vi "AMC_QuickMovePan.vi"(8 "error in (no error)":errorcluster caption="entrée d'erreur (pas d'erreur)", 11 "ConnID":refnum<k5>) -> (0 "error out":errorcluster caption="sortie d'erreur")   [LabVIEW 2019]
uses:
  <vilib>/Utility/config.llb/Read Key (String).vi
  <vilib>/Utility/config.llb/Read Key (U32).vi
  <vilib>/Utility/config.llb/NI_LVConfig.lvlib
panel:
  in  "Ctrl 3":bool
  in  "Ctrl 2":bool
  in  "Ctrl1":bool
  in  "Step3(um)":dbl=0.25 caption="Focus Step(um)"
  in  "Step2(um)":dbl=1.0 caption="Y Step(um)"
  in  "Axis Nm 1":string
  in  "axis3":u8
  in  "Init":bool
  in  "axis1":u8
  in  "axis2":u8
  in  "Axis Nm 3":string
  in  "Axis Nm 2":string
  in  "Up Z":bool
  in  "Down Z":bool
  in  "Quit":bool
  in  "Target 3":dbl=60.0 caption="Focus Target(um)" min=-25000.0 max=25000.0 step=0.001 format="%#.3f"
  out "ActPos 3":dbl=60.0 caption="Focus Act. Pos(um)" min=0.1 step=0.1 format="%#.3f"
  out "ActPos 2":dbl=60.0 caption="Y Act. Pos(um)" min=0.1 step=0.1 format="%#.3f"
  in  "Target 2":dbl=60.0 caption="Y Target(um)" min=-25000.0 max=25000.0 step=0.001 format="%#.3f"
  in  "Target 1":dbl=60.0 caption="X Target(um)" min=-25000.0 max=25000.0 step=0.001 format="%#.3f"
  out "ActPos":dbl=60.0 caption="X Act. Pos(um)" min=0.1 step=0.1 format="%#.3f"
  in  "Right":bool
  in  "Left":bool
  in  "Step1(um)":dbl=1.0 caption="X Step(um)"
  in  "Down":bool
  in  "Up":bool
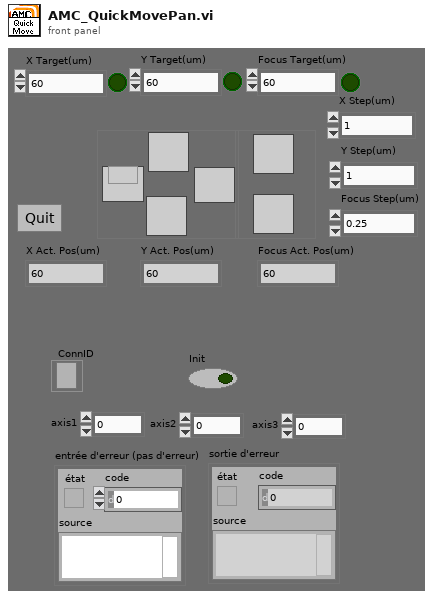
[diagram p1: front panel]
types:
  T1 = enum16{"Répertoire du VI actuel", "Répertoire du parent 1", "Répertoire du parent 2", "Répertoire du parent 3"}
  T2 = typedef "NI_LVConfig.lvlib/Config Data RefNum.ctl" = refnum<k1>
  T3 = typedef "LVRectTypeDef.ctl" = cluster{"Left":i16, "Top":i16, "Right":i16, "Bottom":i16}
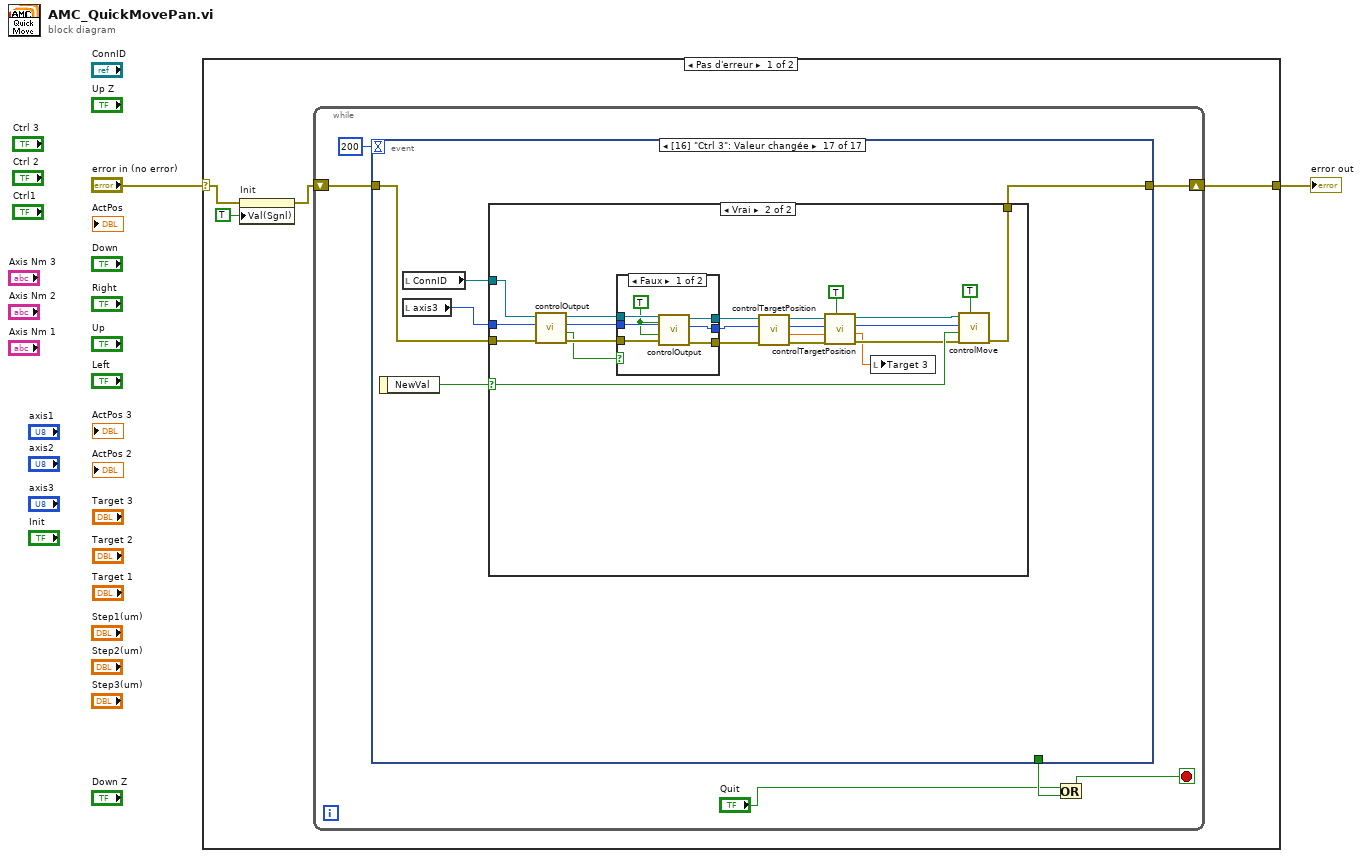
[diagram p0: block diagram]
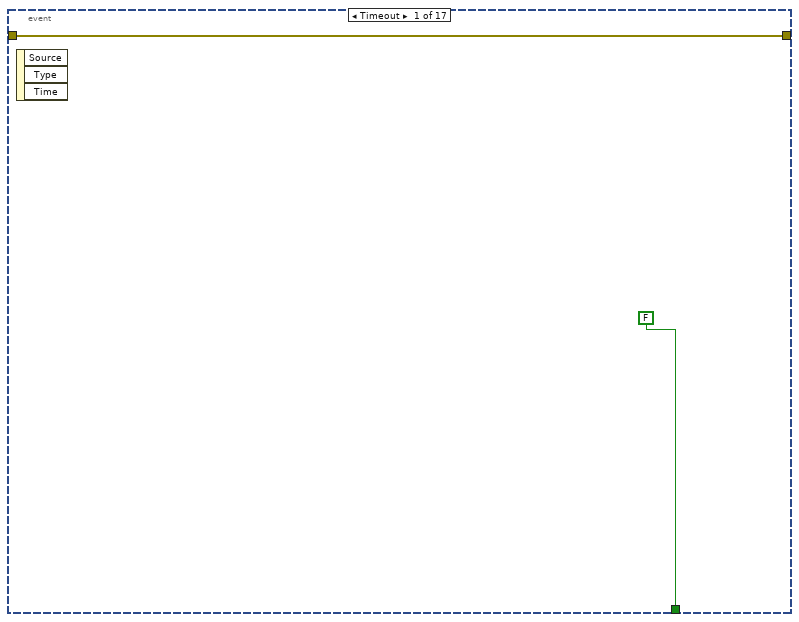
[diagram p2: hidden frame]
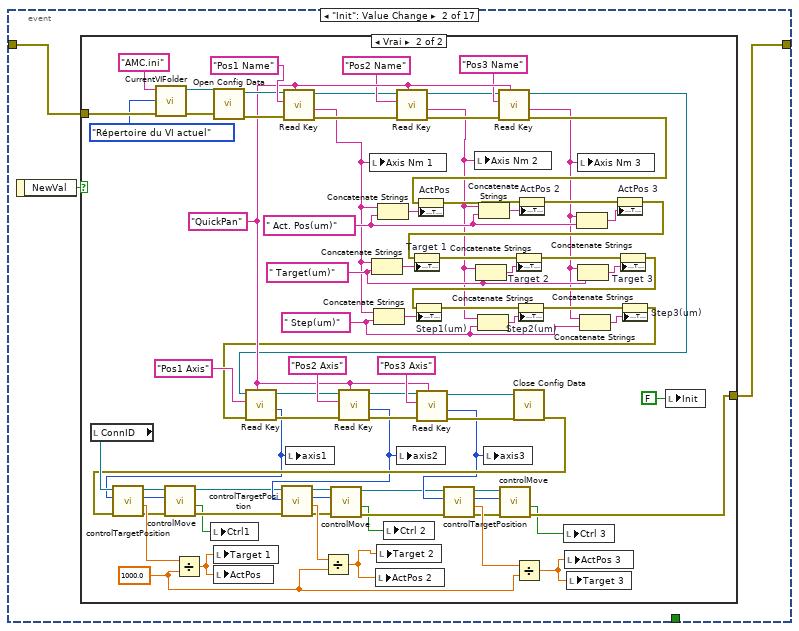
[diagram p3: hidden frame]
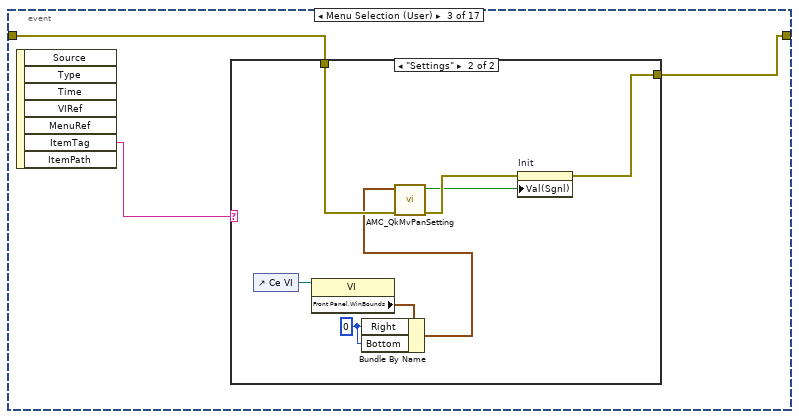
[diagram p5: hidden frame]
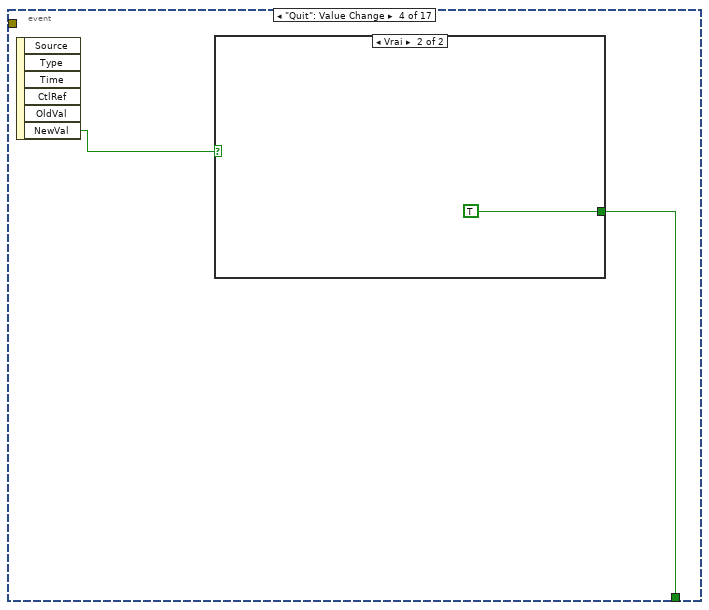
[diagram p7: hidden frame]
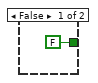
[diagram p8: hidden frame]
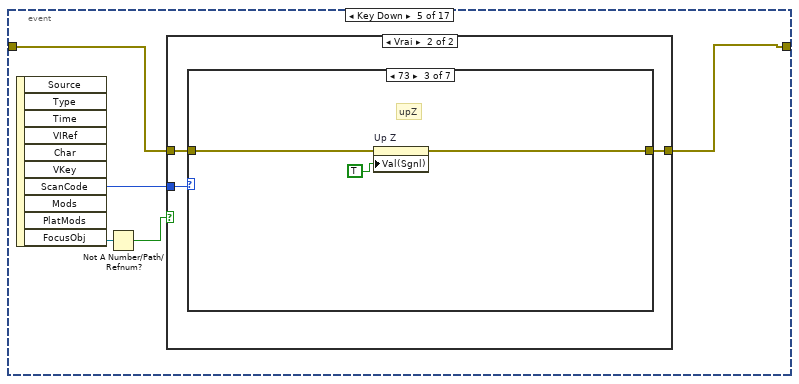
[diagram p9: hidden frame]
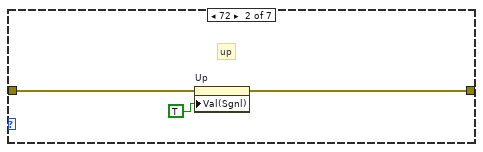
[diagram p12: hidden frame]
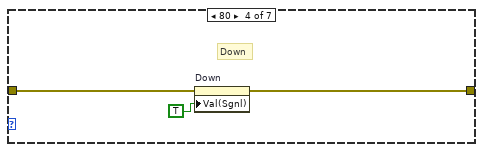
[diagram p13: hidden frame]
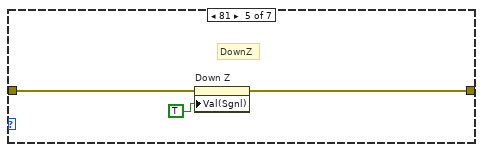
[diagram p14: hidden frame]
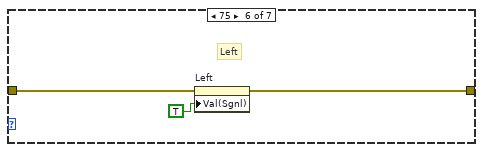
[diagram p15: hidden frame]
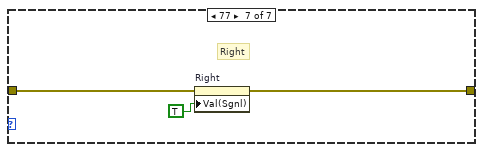
[diagram p16: hidden frame]
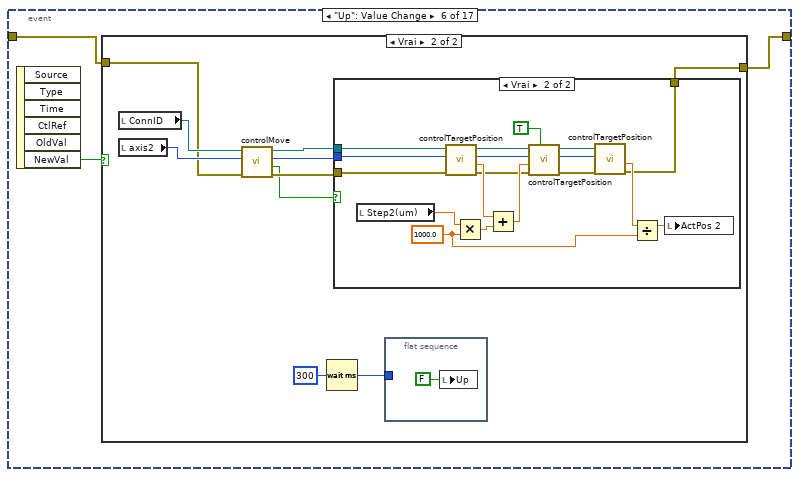
[diagram p17: hidden frame]
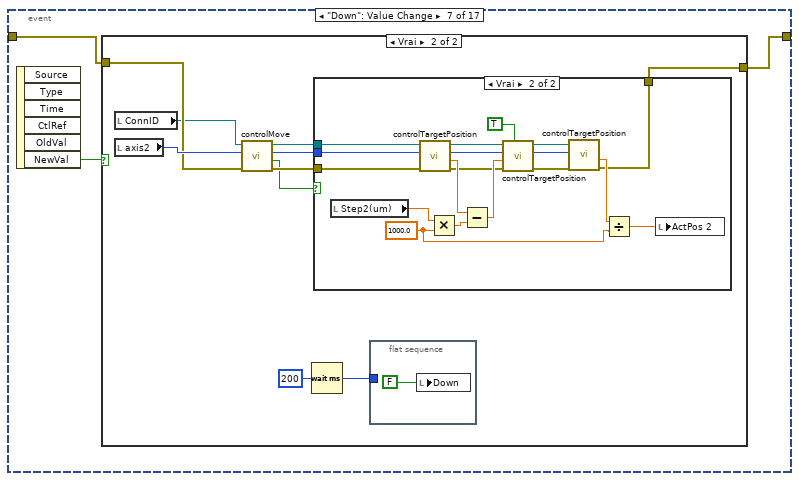
[diagram p20: hidden frame]
diagram:
  n1 = case shown="Pas d'erreur" "error in (no error)" {
    selector: "error in (no error)" -> [w5 w552]
    tunnel: [w6 w552] -> w2
    frame No Error {
      n2 = property on="Init" class="Bool (strict)"(error in=w5, "Val(Sgnl)"=TRUE ("Valeur (Signalisation)")) -> (error out=w4:errorcluster)  [unwired: 1 in, 1 out]
      n3 = while {
        shift-right: [w11] -> w6
        shift-left: w4 -> [w10]
        stop <- w8 stop-if-true
        n4 = event shown="[16] \"Ctrl 3\": Valeur changée" {
          selector: _ -> [_ _ _ _ _ _ _ _ _ _ _ _ _ _ _ _ _]
          dyn-events: _ -> [_ _ _ _ _ _ _ _ _ _ _ _ _ _ _ _ _]
          timeout: 200 -> [_ _ _ _ _ _ _ _ _ _ _ _ _ _ _ _ _]
          tunnel: [w14 w15 w99 _ w118 w143 w177 w211 w245 w279 w313 w356 w382 w407 w423 w466 w509] -> w11
          tunnel: w10 -> [w14 w16 w100 _ w119 w144 w178 w212 w246 w280 w314 w353 w378 w405 w424 w467 w510]
          tunnel: [FALSE _ _ w111 _ _ _ _ _ _ _ _ _ _ _ _ _] -> w9
          event Timeout {
            n5 = event-data() -> ()  [unwired: 1 in, 3 out]
          }
          event "Init": Value Change {
            n6 = event-data() -> ("NewVal"=w17:bool)  [unwired: 1 in]
            n7 = case shown="Vrai" w17 {
              tunnel: w16 -> [w18 w90]
              tunnel: [w18 w22] -> w15
              frame False {
              }
              frame True {
                w42 = 1000.0 ("y")
                w58 = " Step(um)" ("key")
                w59 = " Target(um)" ("key")
                w69 = " Act. Pos(um)" ("key")
                w84 = "QuickPan" ("section")
                n8 = local read "ConnID"() -> (w47:refnum<k5>)
                n9 = call <userlib>:"CurrentVIFolder.vi"("error in (no error)"=w90, "Source"=T1."Répertoire du VI actuel", "NomFichier"="AMC.ini") -> ("error out"=w91:errorcluster, "Chemin"=w92:path)  [unwired: 6 in, 1 out]
                n10 = call <vilib>:"Open Config Data.vi"("error in (no error)"=w91, "configuration file path"=w92) -> ("error out"=w87:errorcluster, "refnum"=w93:T2)  [unwired: 7 in, 1 out]
                n11 = call-poly <vilib>:"Read Key.vi"("section"=w84, "error in (no error)"=w87, "key"="Pos1 Name", "refnum"=w93) -> ("error out"=w86:errorcluster, "value"=w50:string, "refnum out"=w73:T2)  [unwired: 4 in, 1 out]
                n12 = local write "Axis Nm 1"(w50) -> ()
                n13 = Concatenate Strings(w50, w59) -> (w61:string)
                n14 = Concatenate Strings(w50, w58) -> (w57:string)
                n15 = Concatenate Strings(w50, w69) -> (w72:string)
                n16 = call-poly <vilib>:"Read Key.vi"("section"=w84, "error in (no error)"=w86, "key"="Pos2 Name", "refnum"=w73) -> ("error out"=w85:errorcluster, "value"=w49:string, "refnum out"=w74:T2)  [unwired: 4 in, 1 out]
                n17 = local write "Axis Nm 2"(w49) -> ()
                n18 = Concatenate Strings(w49, w59) -> (w62:string)
                n19 = Concatenate Strings(w49, w58) -> (w56:string)
                n20 = Concatenate Strings(w49, w69) -> (w71:string)
                n21 = call-poly <vilib>:"Read Key.vi"("section"=w84, "error in (no error)"=w85, "key"="Pos3 Name", "refnum"=w74) -> ("error out"=w68:errorcluster, "value"=w48:string, "refnum out"=w75:T2)  [unwired: 4 in, 1 out]
                n22 = property on="ActPos" class="NumNb (strict)"(error in=w68, "Caption.Text"=w72) -> (error out=w67:errorcluster)  [unwired: 1 in, 1 out]
                n23 = property on="ActPos 2" class="NumNb (strict)"(error in=w67, "Caption.Text"=w71) -> (error out=w66:errorcluster)  [unwired: 1 in, 1 out]
                n24 = Concatenate Strings(w48, w69) -> (w70:string)
                n25 = local write "Axis Nm 3"(w48) -> ()
                n26 = Concatenate Strings(w48, w59) -> (w63:string)
                n27 = Concatenate Strings(w48, w58) -> (w55:string)
                n28 = property on="ActPos 3" class="NumNb (strict)"(error in=w66, "Caption.Text"=w70) -> (error out=w60:errorcluster)  [unwired: 1 in, 1 out]
                n29 = property on="Target 1" class="NumNb (strict)"(error in=w60, "Caption.Text"=w61) -> (error out=w64:errorcluster)  [unwired: 1 in, 1 out]
                n30 = property on="Target 2" class="NumNb (strict)"(error in=w64, "Caption.Text"=w62) -> (error out=w65:errorcluster)  [unwired: 1 in, 1 out]
                n31 = property on="Target 3" class="NumNb (strict)"(error in=w65, "Caption.Text"=w63) -> (error out=w51:errorcluster)  [unwired: 1 in, 1 out]
                n32 = property on="Step1(um)" class="NumNb (strict)"(error in=w51, "Caption.Text"=w57) -> (error out=w54:errorcluster)  [unwired: 1 in, 1 out]
                n33 = property on="Step2(um)" class="NumNb (strict)"(error in=w54, "Caption.Text"=w56) -> (error out=w53:errorcluster)  [unwired: 1 in, 1 out]
                n34 = property on="Step3(um)" class="NumNb (strict)"(error in=w53, "Caption.Text"=w55) -> (error out=w52:errorcluster)  [unwired: 1 in, 1 out]
                n35 = call-poly <vilib>:"Read Key.vi"("section"=w84, "error in (no error)"=w52, "key"="Pos1 Axis", "refnum"=w75) -> ("error out"=w77:errorcluster, "value"=w39:u32, "refnum out"=w81:T2)  [unwired: 4 in, 1 out]
                n36 = local write "axis1"(w39) -> ()
                n37 = call-poly <vilib>:"Read Key.vi"("section"=w84, "error in (no error)"=w77, "key"="Pos2 Axis", "refnum"=w81) -> ("error out"=w76:errorcluster, "value"=w38:u32, "refnum out"=w80:T2)  [unwired: 4 in, 1 out]
                n38 = local write "axis2"(w38) -> ()
                n39 = call-poly <vilib>:"Read Key.vi"("section"=w84, "error in (no error)"=w76, "key"="Pos3 Axis", "refnum"=w80) -> ("error out"=w78:errorcluster, "value"=w37:u32, "refnum out"=w79:T2)  [unwired: 4 in, 1 out]
                n40 = local write "axis3"(w37) -> ()
                n41 = call <vilib>:"Close Config Data.vi"("error in (no error)"=w78, "refnum"=w79) -> ("error out"=w46:errorcluster)  [unwired: 8 in, 1 out]
                n42 = call <userlib>:"controlTargetPosition.vi"("error in"=w46, "axis in"=w39, "connection ID"=w47) -> ("error out"=w34:errorcluster, "Target Position out"=w36:dbl, "axis out"=w33:u8, "connection ID"=w35:refnum<k5>)  [unwired: 5 in]
                n43 = call <userlib>:"controlMove.vi"("error in"=w34, "axis in"=w33, "connection ID"=w35) -> ("error out"=w26:errorcluster, "controll move out"=w21:bool, "connection ID"=w25:refnum<k5>)  [unwired: 5 in, 1 out]
                n44 = Divide(x=w36, y=w42) -> (x/y=w44:dbl)
                n45 = local write "Ctrl1"(w21) -> ()
                n46 = local write "Target 1"(w44) -> ()
                n47 = local write "ActPos"(w44) -> ()
                n48 = call <userlib>:"controlTargetPosition.vi"("error in"=w26, "axis in"=w38, "connection ID"=w25) -> ("error out"=w32:errorcluster, "Target Position out"=w45:dbl, "axis out"=w30:u8, "connection ID"=w31:refnum<k5>)  [unwired: 5 in]
                n49 = Divide(x=w45, y=w42) -> (x/y=w43:dbl)
                n50 = call <userlib>:"controlMove.vi"("error in"=w32, "axis in"=w30, "connection ID"=w31) -> ("error out"=w23:errorcluster, "controll move out"=w19:bool, "connection ID"=w24:refnum<k5>)  [unwired: 5 in, 1 out]
                n51 = local write "ActPos 2"(w43) -> ()
                n52 = local write "Target 2"(w43) -> ()
                n53 = local write "Ctrl 2"(w19) -> ()
                n54 = call <userlib>:"controlTargetPosition.vi"("error in"=w23, "axis in"=w37, "connection ID"=w24) -> ("error out"=w29:errorcluster, "Target Position out"=w41:dbl, "axis out"=w27:u8, "connection ID"=w28:refnum<k5>)  [unwired: 5 in]
                n55 = call <userlib>:"controlMove.vi"("error in"=w29, "axis in"=w27, "connection ID"=w28) -> ("error out"=w22:errorcluster, "controll move out"=w20:bool)  [unwired: 5 in, 2 out]
                n56 = Divide(x=w41, y=w42) -> (x/y=w40:dbl)
                n57 = local write "Ctrl 3"(w20) -> ()
                n58 = local write "ActPos 3"(w40) -> ()
                n59 = local write "Target 3"(w40) -> ()
                n60 = local write "Init"(FALSE ("Init")) -> ()
              }
            }
          }
          event Menu Selection (User) {
            n61 = event-data() -> ("ItemTag"=w101:string)  [unwired: 1 in, 6 out]
            n62 = case shown="\"Settings\"" w101 {
              tunnel: w100 -> [w102 w109]
              tunnel: [w102 w110] -> w99
              frame Default {
              }
              frame "Settings" {
                w104 = i16 0 ("Right")
                n63 = control-ref of="Ce VI"() -> (w106:refnum<vi>)
                n64 = property class="VI"(reference=w106) -> ("Front Panel.WinBounds"=w105:T3)  [unwired: 1 in, 2 out]
                n65 = Bundle By Name(cluster=w105, "Right"=w104, "Bottom"=w104) -> (w103:T3)
                n66 = call <userlib>:"AMC_QkMvPanSetting.vi"("error in (no error)"=w109, "Fenêtre face-avant:Limites"=w103) -> ("error out"=w108:errorcluster, "Saved set"=w107:bool)  [unwired: 8 in]
                n67 = property on="Init" class="Bool (strict)"(error in=w108, "Val(Sgnl)"=w107) -> (error out=w110:errorcluster)  [unwired: 1 in, 1 out]
              }
            }
          }
          event "Quit": Value Change {
            n68 = event-data() -> ("NewVal"=w112:bool)  [unwired: 1 in, 5 out]
            n69 = case shown="Vrai" w112 {
              tunnel: [FALSE TRUE] -> w111
              frame False {
              }
              frame True {
              }
            }
          }
          event Key Down {
            n70 = event-data() -> ("ScanCode"=w115:i16, "FocusObj"=w117:refnum<vi>)  [unwired: 1 in, 8 out]
            n71 = Not A Number/Path/Refnum?(number/path/refnum=w117) -> (NaN/Path/Refnum?=w116:bool)
            n72 = case shown="Vrai" w116 {
              tunnel: w115 -> [_ w123]
              tunnel: w119 -> [w120 w122]
              tunnel: [w120 w121] -> w118
              frame False {
              }
              frame True {
                n73 = case shown="73" w123 {
                  tunnel: w122 -> [w124 w127 w130 w133 w136 w139 w142]
                  tunnel: [w124 w126 w129 w132 w135 w138 w141] -> w121
                  frame 0, Default {
                  }
                  frame 72 {
                    # "up"
                    n74 = property on="Up" class="Bool (strict)"(error in=w127, "Val(Sgnl)"=TRUE) -> (error out=w126:errorcluster)  [unwired: 1 in, 1 out]
                  }
                  frame 73 {
                    # "upZ"
                    n75 = property on="Up Z" class="Bool (strict)"(error in=w130, "Val(Sgnl)"=TRUE) -> (error out=w129:errorcluster)  [unwired: 1 in, 1 out]
                  }
                  frame 80 {
                    # "Down"
                    n76 = property on="Down" class="Bool (strict)"(error in=w133, "Val(Sgnl)"=TRUE) -> (error out=w132:errorcluster)  [unwired: 1 in, 1 out]
                  }
                  frame 81 {
                    # "DownZ"
                    n77 = property on="Down Z" class="Bool (strict)"(error in=w136, "Val(Sgnl)"=TRUE) -> (error out=w135:errorcluster)  [unwired: 1 in, 1 out]
                  }
                  frame 75 {
                    # "Left"
                    n78 = property on="Left" class="Bool (strict)"(error in=w139, "Val(Sgnl)"=TRUE) -> (error out=w138:errorcluster)  [unwired: 1 in, 1 out]
                  }
                  frame 77 {
                    # "Right"
                    n79 = property on="Right" class="Bool (strict)"(error in=w142, "Val(Sgnl)"=TRUE) -> (error out=w141:errorcluster)  [unwired: 1 in, 1 out]
                  }
                }
              }
            }
          }
          event "Up": Value Change {
            n80 = event-data() -> ("NewVal"=w145:bool)  [unwired: 1 in, 5 out]
            n81 = case shown="Vrai" w145 {
              tunnel: w144 -> [w146 w151]
              tunnel: [w146 w154] -> w143
              frame False {
              }
              frame True {
                n82 = local read "ConnID"() -> (w153:refnum<k5>)
                n83 = local read "axis2"() -> (w152:u8)
                n84 = call <userlib>:"controlMove.vi"("error in"=w151, "axis in"=w152, "connection ID"=w153) -> ("error out"=w150:errorcluster, "controll move out"=w147:bool, "axis out"=w149:u8, "connection ID"=w148:refnum<k5>)  [unwired: 5 in]
                n85 = Wait (ms)(milliseconds to wait=u32 300 ("attente (ms)")) -> (millisecond timer value=w156:u32)
                n86 = case shown="Vrai" w147 {
                  tunnel: w150 -> [w157 w169]
                  tunnel: [w157 w166] -> w154
                  tunnel: w149 -> [_ w164]
                  tunnel: w148 -> [_ w160]
                  frame False {
                  }
                  frame True {
                    w158 = 1000.0 ("y")
                    n87 = local read "Step2(um)"() -> (w172:dbl)
                    n88 = call <userlib>:"controlTargetPosition.vi"("error in"=w169, "axis in"=w164, "connection ID"=w160) -> ("error out"=w170:errorcluster, "Target Position out"=w174:dbl, "axis out"=w175:u8, "connection ID"=w162:refnum<k5>)  [unwired: 5 in]
                    n89 = Multiply(x=w172, y=w158) -> (x*y=w173:dbl)
                    n90 = Add(x=w174, y=w173) -> (x+y=w171:dbl)
                    n91 = call <userlib>:"controlTargetPosition.vi"("Set"=TRUE, "error in"=w170, "Target Position in"=w171, "axis in"=w175, "connection ID"=w162) -> ("error out"=w168:errorcluster, "axis out"=w165:u8, "connection ID"=w161:refnum<k5>)  [unwired: 3 in, 1 out]
                    n92 = call <userlib>:"controlTargetPosition.vi"("error in"=w168, "axis in"=w165, "connection ID"=w161) -> ("error out"=w166:errorcluster, "Target Position out"=w167:dbl)  [unwired: 5 in, 2 out]
                    n93 = Divide(x=w167, y=w158) -> (x/y=w159:dbl)
                    n94 = local write "ActPos 2"(w159) -> ()
                  }
                }
                n95 = flat-sequence {
                  tunnel: w156 -> [_]
                  frame #0 {
                    n96 = local write "Up"(FALSE ("Up")) -> ()
                  }
                }
              }
            }
          }
          event "Down": Value Change {
            n97 = event-data() -> ("NewVal"=w179:bool)  [unwired: 1 in, 5 out]
            n98 = case shown="Vrai" w179 {
              tunnel: w178 -> [w180 w186]
              tunnel: [w180 w188] -> w177
              frame False {
              }
              frame True {
                n99 = local read "ConnID"() -> (w183:refnum<k5>)
                n100 = local read "axis2"() -> (w187:u8)
                n101 = call <userlib>:"controlMove.vi"("error in"=w186, "axis in"=w187, "connection ID"=w183) -> ("error out"=w185:errorcluster, "controll move out"=w181:bool, "axis out"=w184:u8, "connection ID"=w182:refnum<k5>)  [unwired: 5 in]
                n102 = Wait (ms)(milliseconds to wait=u32 200 ("attente (ms)")) -> (millisecond timer value=w190:u32)
                n103 = case shown="Vrai" w181 {
                  tunnel: [w191 w201] -> w188
                  tunnel: w185 -> [w191 w194]
                  tunnel: w184 -> [_ w193]
                  tunnel: w182 -> [_ w192]
                  frame False {
                  }
                  frame True {
                    w195 = 1000.0 ("y")
                    n104 = local read "Step2(um)"() -> (w206:dbl)
                    n105 = call <userlib>:"controlTargetPosition.vi"("error in"=w194, "axis in"=w193, "connection ID"=w192) -> ("error out"=w204:errorcluster, "Target Position out"=w208:dbl, "axis out"=w209:u8, "connection ID"=w198:refnum<k5>)  [unwired: 5 in]
                    n106 = Multiply(x=w206, y=w195) -> (x*y=w207:dbl)
                    n107 = Subtract(x=w208, y=w207) -> (x-y=w205:dbl)
                    n108 = call <userlib>:"controlTargetPosition.vi"("Set"=TRUE, "error in"=w204, "Target Position in"=w205, "axis in"=w209, "connection ID"=w198) -> ("error out"=w203:errorcluster, "axis out"=w200:u8, "connection ID"=w197:refnum<k5>)  [unwired: 3 in, 1 out]
                    n109 = call <userlib>:"controlTargetPosition.vi"("error in"=w203, "axis in"=w200, "connection ID"=w197) -> ("error out"=w201:errorcluster, "Target Position out"=w202:dbl)  [unwired: 5 in, 2 out]
                    n110 = Divide(x=w202, y=w195) -> (x/y=w196:dbl)
                    n111 = local write "ActPos 2"(w196) -> ()
                  }
                }
                n112 = flat-sequence {
                  tunnel: w190 -> [_]
                  frame #0 {
                    n113 = local write "Down"(FALSE ("Up")) -> ()
                  }
                }
              }
            }
          }
          event "Left": Value Change {
            n114 = event-data() -> ("NewVal"=w213:bool)  [unwired: 1 in, 5 out]
            n115 = case shown="Vrai" w213 {
              tunnel: w212 -> [w214 w221]
              tunnel: [w214 w222] -> w211
              frame False {
              }
              frame True {
                n116 = local read "ConnID"() -> (w220:refnum<k5>)
                n117 = local read "axis1"() -> (w219:u8)
                n118 = call <userlib>:"controlMove.vi"("error in"=w221, "axis in"=w219, "connection ID"=w220) -> ("error out"=w218:errorcluster, "controll move out"=w215:bool, "axis out"=w217:u8, "connection ID"=w216:refnum<k5>)  [unwired: 5 in]
                n119 = case shown="Vrai" w215 {
                  tunnel: w218 -> [w225 w237]
                  tunnel: [w225 w234] -> w222
                  tunnel: w217 -> [_ w232]
                  tunnel: w216 -> [_ w228]
                  frame False {
                  }
                  frame True {
                    w226 = 1000.0 ("y")
                    n120 = local read "Step1(um)"() -> (w240:dbl)
                    n121 = call <userlib>:"controlTargetPosition.vi"("error in"=w237, "axis in"=w232, "connection ID"=w228) -> ("error out"=w238:errorcluster, "Target Position out"=w242:dbl, "axis out"=w243:u8, "connection ID"=w230:refnum<k5>)  [unwired: 5 in]
                    n122 = Multiply(x=w240, y=w226) -> (x*y=w241:dbl)
                    n123 = Subtract(x=w242, y=w241) -> (x-y=w239:dbl)
                    n124 = call <userlib>:"controlTargetPosition.vi"("Set"=TRUE, "error in"=w238, "Target Position in"=w239, "axis in"=w243, "connection ID"=w230) -> ("error out"=w236:errorcluster, "axis out"=w233:u8, "connection ID"=w229:refnum<k5>)  [unwired: 3 in, 1 out]
                    n125 = call <userlib>:"controlTargetPosition.vi"("error in"=w236, "axis in"=w233, "connection ID"=w229) -> ("error out"=w234:errorcluster, "Target Position out"=w235:dbl)  [unwired: 5 in, 2 out]
                    n126 = Divide(x=w235, y=w226) -> (x/y=w227:dbl)
                    n127 = local write "ActPos"(w227) -> ()
                  }
                }
                n128 = Wait (ms)(milliseconds to wait=u32 200 ("attente (ms)")) -> (millisecond timer value=w224:u32)
                n129 = flat-sequence {
                  tunnel: w224 -> [_]
                  frame #0 {
                    n130 = local write "Left"(FALSE ("Up")) -> ()
                  }
                }
              }
            }
          }
          event "Right": Value Change {
            n131 = event-data() -> ("NewVal"=w247:bool)  [unwired: 1 in, 5 out]
            n132 = case shown="Vrai" w247 {
              tunnel: w246 -> [w248 w255]
              tunnel: [w248 w256] -> w245
              frame False {
              }
              frame True {
                n133 = local read "ConnID"() -> (w253:refnum<k5>)
                n134 = local read "axis1"() -> (w254:u8)
                n135 = call <userlib>:"controlMove.vi"("error in"=w255, "axis in"=w254, "connection ID"=w253) -> ("error out"=w250:errorcluster, "controll move out"=w249:bool, "axis out"=w252:u8, "connection ID"=w251:refnum<k5>)  [unwired: 5 in]
                n136 = case shown="Vrai" w249 {
                  tunnel: w250 -> [w259 w271]
                  tunnel: [w259 w268] -> w256
                  tunnel: w252 -> [_ w266]
                  tunnel: w251 -> [_ w262]
                  frame False {
                  }
                  frame True {
                    w260 = 1000.0 ("y")
                    n137 = local read "Step1(um)"() -> (w274:dbl)
                    n138 = call <userlib>:"controlTargetPosition.vi"("error in"=w271, "axis in"=w266, "connection ID"=w262) -> ("error out"=w272:errorcluster, "Target Position out"=w276:dbl, "axis out"=w277:u8, "connection ID"=w264:refnum<k5>)  [unwired: 5 in]
                    n139 = Multiply(x=w274, y=w260) -> (x*y=w275:dbl)
                    n140 = Add(x=w276, y=w275) -> (x+y=w273:dbl)
                    n141 = call <userlib>:"controlTargetPosition.vi"("Set"=TRUE, "error in"=w272, "Target Position in"=w273, "axis in"=w277, "connection ID"=w264) -> ("error out"=w270:errorcluster, "axis out"=w267:u8, "connection ID"=w263:refnum<k5>)  [unwired: 3 in, 1 out]
                    n142 = call <userlib>:"controlTargetPosition.vi"("error in"=w270, "axis in"=w267, "connection ID"=w263) -> ("error out"=w268:errorcluster, "Target Position out"=w269:dbl)  [unwired: 5 in, 2 out]
                    n143 = Divide(x=w269, y=w260) -> (x/y=w261:dbl)
                    n144 = local write "ActPos"(w261) -> ()
                  }
                }
                n145 = Wait (ms)(milliseconds to wait=u32 200 ("attente (ms)")) -> (millisecond timer value=w258:u32)
                n146 = flat-sequence {
                  tunnel: w258 -> [_]
                  frame #0 {
                    n147 = local write "Right"(FALSE ("Up")) -> ()
                  }
                }
              }
            }
          }
          event "Down Z": Value Change {
            n148 = event-data() -> ("NewVal"=w281:bool)  [unwired: 1 in, 5 out]
            n149 = case shown="Vrai" w281 {
              tunnel: w280 -> [w282 w287]
              tunnel: [w282 w290] -> w279
              frame False {
              }
              frame True {
                n150 = local read "axis3"() -> (w288:u8)
                n151 = local read "ConnID"() -> (w289:refnum<k5>)
                n152 = call <userlib>:"controlMove.vi"("error in"=w287, "axis in"=w288, "connection ID"=w289) -> ("error out"=w286:errorcluster, "controll move out"=w285:bool, "axis out"=w283:u8, "connection ID"=w284:refnum<k5>)  [unwired: 5 in]
                n153 = case shown="Vrai" w285 {
                  tunnel: [w293 w303] -> w290
                  tunnel: w286 -> [w293 w296]
                  tunnel: w284 -> [_ w295]
                  tunnel: w283 -> [_ w294]
                  frame False {
                  }
                  frame True {
                    w297 = 1000.0 ("y")
                    n154 = local read "Step3(um)"() -> (w308:dbl)
                    n155 = call <userlib>:"controlTargetPosition.vi"("error in"=w296, "axis in"=w294, "connection ID"=w295) -> ("error out"=w306:errorcluster, "Target Position out"=w310:dbl, "axis out"=w311:u8, "connection ID"=w300:refnum<k5>)  [unwired: 5 in]
                    n156 = Multiply(x=w308, y=w297) -> (x*y=w309:dbl)
                    n157 = Subtract(x=w310, y=w309) -> (x-y=w307:dbl)
                    n158 = call <userlib>:"controlTargetPosition.vi"("Set"=TRUE, "error in"=w306, "Target Position in"=w307, "axis in"=w311, "connection ID"=w300) -> ("error out"=w305:errorcluster, "axis out"=w302:u8, "connection ID"=w299:refnum<k5>)  [unwired: 3 in, 1 out]
                    n159 = call <userlib>:"controlTargetPosition.vi"("error in"=w305, "axis in"=w302, "connection ID"=w299) -> ("error out"=w303:errorcluster, "Target Position out"=w304:dbl)  [unwired: 5 in, 2 out]
                    n160 = Divide(x=w304, y=w297) -> (x/y=w298:dbl)
                    n161 = local write "ActPos 3"(w298) -> ()
                  }
                }
                n162 = Wait (ms)(milliseconds to wait=u32 200 ("attente (ms)")) -> (millisecond timer value=w292:u32)
                n163 = flat-sequence {
                  tunnel: w292 -> [_]
                  frame #0 {
                    n164 = local write "Down Z"(FALSE ("Up")) -> ()
                  }
                }
              }
            }
          }
          event "Up Z": Value Change {
            n165 = event-data() -> ("NewVal"=w315:bool)  [unwired: 1 in, 5 out]
            n166 = case shown="Vrai" w315 {
              tunnel: w314 -> [w316 w318]
              tunnel: [w316 w324] -> w313
              frame False {
              }
              frame True {
                n167 = local read "ConnID"() -> (w320:refnum<k5>)
                n168 = local read "axis3"() -> (w319:u8)
                n169 = call <userlib>:"controlMove.vi"("error in"=w318, "axis in"=w319, "connection ID"=w320) -> ("error out"=w323:errorcluster, "controll move out"=w317:bool, "axis out"=w322:u8, "connection ID"=w321:refnum<k5>)  [unwired: 5 in]
                n170 = case shown="Vrai" w317 {
                  tunnel: w323 -> [w327 w339]
                  tunnel: [w327 w336] -> w324
                  tunnel: w322 -> [_ w334]
                  tunnel: w321 -> [_ w330]
                  frame False {
                  }
                  frame True {
                    w328 = 1000.0 ("y")
                    n171 = local read "Step3(um)"() -> (w342:dbl)
                    n172 = call <userlib>:"controlTargetPosition.vi"("error in"=w339, "axis in"=w334, "connection ID"=w330) -> ("error out"=w340:errorcluster, "Target Position out"=w344:dbl, "axis out"=w345:u8, "connection ID"=w332:refnum<k5>)  [unwired: 5 in]
                    n173 = Multiply(x=w342, y=w328) -> (x*y=w343:dbl)
                    n174 = Add(x=w344, y=w343) -> (x+y=w341:dbl)
                    n175 = call <userlib>:"controlTargetPosition.vi"("Set"=TRUE, "error in"=w340, "Target Position in"=w341, "axis in"=w345, "connection ID"=w332) -> ("error out"=w338:errorcluster, "axis out"=w335:u8, "connection ID"=w331:refnum<k5>)  [unwired: 3 in, 1 out]
                    n176 = call <userlib>:"controlTargetPosition.vi"("error in"=w338, "axis in"=w335, "connection ID"=w331) -> ("error out"=w336:errorcluster, "Target Position out"=w337:dbl)  [unwired: 5 in, 2 out]
                    n177 = Divide(x=w337, y=w328) -> (x/y=w329:dbl)
                    n178 = local write "ActPos 3"(w329) -> ()
                  }
                }
                n179 = Wait (ms)(milliseconds to wait=u32 200 ("attente (ms)")) -> (millisecond timer value=w326:u32)
                n180 = flat-sequence {
                  tunnel: w326 -> [_]
                  frame #0 {
                    n181 = local write "Up Z"(FALSE ("Up")) -> ()
                  }
                }
              }
            }
          }
          event "Target 1": Value Change {
            n182 = event-data() -> ("NewVal"=w355:dbl)  [unwired: 1 in, 5 out]
            n183 = local read "ConnID"() -> (w352:refnum<k5>)
            n184 = local read "axis1"() -> (w351:u8)
            n185 = call <userlib>:"controlMove.vi"("error in"=w353, "axis in"=w351, "connection ID"=w352) -> ("error out"=w354:errorcluster, "controll move out"=w348:bool, "axis out"=w349:u8, "connection ID"=w350:refnum<k5>)  [unwired: 5 in]
            n186 = case shown="Faux" w348 {
              tunnel: [w357 w371] -> w356
              tunnel: w355 -> [w358 w363]
              tunnel: w354 -> [w357 w362]
              tunnel: w350 -> [_ w361]
              tunnel: w349 -> [_ w360]
              tunnel: [w358 w359] -> w347
              frame False {
              }
              frame True {
                w365 = 1000.0 ("y")
                n187 = Multiply(x=w363, y=w365) -> (x*y=w364:dbl)
                n188 = call <userlib>:"controlTargetPosition.vi"("Set"=TRUE, "error in"=w362, "Target Position in"=w364, "axis in"=w360, "connection ID"=w361) -> ("error out"=w370:errorcluster, "axis out"=w368:u8, "connection ID"=w366:refnum<k5>)  [unwired: 3 in, 1 out]
                n189 = call <userlib>:"controlTargetPosition.vi"("error in"=w370, "axis in"=w368, "connection ID"=w366) -> ("error out"=w371:errorcluster, "Target Position out"=w369:dbl)  [unwired: 5 in, 2 out]
                n190 = Divide(x=w369, y=w365) -> (x/y=w359:dbl)
              }
            }
            n191 = local write "ActPos"(w347) -> ()
          }
          event "Target 2": Value Change {
            n192 = event-data() -> ("OldVal"=w372:dbl, "NewVal"=w381:dbl)  [unwired: 1 in, 4 out]
            n193 = local read "ConnID"() -> (w380:refnum<k5>)
            n194 = local read "axis2"() -> (w379:u8)
            n195 = call <userlib>:"controlMove.vi"("error in"=w378, "axis in"=w379, "connection ID"=w380) -> ("error out"=w375:errorcluster, "controll move out"=w374:bool, "axis out"=w376:u8, "connection ID"=w377:refnum<k5>)  [unwired: 5 in]
            n196 = case shown="Vrai" w374 {
              tunnel: [w384 w397] -> w382
              tunnel: w381 -> [_ w391]
              tunnel: w377 -> [_ w388]
              tunnel: w376 -> [_ w387]
              tunnel: w375 -> [w384 w386]
              tunnel: [w383 w385] -> w373
              tunnel: w372 -> [w383 _]
              frame False {
              }
              frame True {
                w389 = 1000.0 ("y")
                n197 = Multiply(x=w391, y=w389) -> (x*y=w390:dbl)
                n198 = call <userlib>:"controlTargetPosition.vi"("Set"=TRUE, "error in"=w386, "Target Position in"=w390, "axis in"=w387, "connection ID"=w388) -> ("error out"=w396:errorcluster, "axis out"=w394:u8, "connection ID"=w392:refnum<k5>)  [unwired: 3 in, 1 out]
                n199 = call <userlib>:"controlTargetPosition.vi"("error in"=w396, "axis in"=w394, "connection ID"=w392) -> ("error out"=w397:errorcluster, "Target Position out"=w395:dbl)  [unwired: 5 in, 2 out]
                n200 = Divide(x=w395, y=w389) -> (x/y=w385:dbl)
              }
            }
            n201 = local write "ActPos 2"(w373) -> ()
          }
          event "Target 3": Value Change {
            n202 = event-data() -> ("NewVal"=w406:dbl)  [unwired: 1 in, 5 out]
            n203 = local read "ConnID"() -> (w403:refnum<k5>)
            n204 = local read "axis3"() -> (w404:u8)
            n205 = call <userlib>:"controlMove.vi"("error in"=w405, "axis in"=w404, "connection ID"=w403) -> ("error out"=w400:errorcluster, "controll move out"=w399:bool, "axis out"=w402:u8, "connection ID"=w401:refnum<k5>)  [unwired: 5 in]
            n206 = case shown="Vrai" w399 {
              tunnel: [w408 w422] -> w407
              tunnel: w406 -> [w409 w416]
              tunnel: w402 -> [_ w413]
              tunnel: w401 -> [_ w412]
              tunnel: w400 -> [w408 w411]
              tunnel: [w409 w410] -> w398
              frame False {
              }
              frame True {
                w414 = 1000.0 ("y")
                n207 = Multiply(x=w416, y=w414) -> (x*y=w415:dbl)
                n208 = call <userlib>:"controlTargetPosition.vi"("Set"=TRUE, "error in"=w411, "Target Position in"=w415, "axis in"=w413, "connection ID"=w412) -> ("error out"=w421:errorcluster, "axis out"=w419:u8, "connection ID"=w417:refnum<k5>)  [unwired: 3 in, 1 out]
                n209 = call <userlib>:"controlTargetPosition.vi"("error in"=w421, "axis in"=w419, "connection ID"=w417) -> ("error out"=w422:errorcluster, "Target Position out"=w420:dbl)  [unwired: 5 in, 2 out]
                n210 = Divide(x=w420, y=w414) -> (x/y=w410:dbl)
              }
            }
            n211 = local write "ActPos 3"(w398) -> ()
          }
          event "Ctrl1": Value Change {
            n212 = event-data() -> ("NewVal"=w427:bool)  [unwired: 1 in]
            n213 = local read "ConnID"() -> (w425:refnum<k5>)
            n214 = local read "axis1"() -> (w426:u8)
            n215 = case shown="Faux" w427 {
              selector: w427 -> [w428 w454]
              tunnel: w425 -> [w430 w441]
              tunnel: w426 -> [w431 w442]
              tunnel: w424 -> [w432 w443]
              tunnel: [w429 w444] -> w423
              frame False {
                n216 = call <userlib>:"controlMove.vi"("Set"=TRUE, "error in"=w432, "control move in"=w428, "axis in"=w431, "connection ID"=w430) -> ("error out"=w429:errorcluster)  [unwired: 3 in, 3 out]
              }
              frame True {
                n217 = call <userlib>:"controlOutput.vi"("error in"=w443, "axis in"=w442, "connection ID"=w441) -> ("error out"=w440:errorcluster, "enable output out"=w439:bool, "axis out"=w436:u8, "connection ID"=w437:refnum<k5>)  [unwired: 5 in]
                n218 = case shown="Faux" w439 {
                  tunnel: w440 -> [w462 w465]
                  tunnel: [w461 w465] -> w438
                  tunnel: w437 -> [w460 w464]
                  tunnel: w436 -> [w459 w463]
                  tunnel: [w458 w464] -> w435
                  tunnel: [w457 w463] -> w434
                  frame False {
                    w456 = TRUE ("Set")
                    n219 = call <userlib>:"controlOutput.vi"("Set"=w456, "error in"=w462, "enable output in"=w456, "axis in"=w459, "connection ID"=w460) -> ("error out"=w461:errorcluster, "axis out"=w457:u8, "connection ID"=w458:refnum<k5>)  [unwired: 3 in, 1 out]
                  }
                  frame True {
                  }
                }
                n220 = call <userlib>:"controlTargetPosition.vi"("error in"=w438, "axis in"=w434, "connection ID"=w435) -> ("error out"=w453:errorcluster, "Target Position out"=w446:dbl, "axis out"=w452:u8, "connection ID"=w451:refnum<k5>)  [unwired: 5 in]
                n221 = call <userlib>:"controlTargetPosition.vi"("Set"=TRUE, "error in"=w453, "Target Position in"=w446, "axis in"=w452, "connection ID"=w451) -> ("error out"=w449:errorcluster, "Target Position out"=w445:dbl, "axis out"=w447:u8, "connection ID"=w448:refnum<k5>)  [unwired: 3 in]
                n222 = local write "Target 1"(w445) -> ()
                n223 = call <userlib>:"controlMove.vi"("Set"=TRUE, "error in"=w449, "control move in"=w454, "axis in"=w447, "connection ID"=w448) -> ("error out"=w444:errorcluster)  [unwired: 3 in, 3 out]
              }
            }
          }
          event "Ctrl 2": Value Change {
            n224 = event-data() -> ("NewVal"=w470:bool)  [unwired: 1 in]
            n225 = local read "ConnID"() -> (w468:refnum<k5>)
            n226 = local read "axis2"() -> (w469:u8)
            n227 = case shown="Vrai" w470 {
              selector: w470 -> [w471 w497]
              tunnel: w468 -> [w473 w484]
              tunnel: w469 -> [w474 w485]
              tunnel: w467 -> [w475 w486]
              tunnel: [w472 w487] -> w466
              frame False {
                n228 = call <userlib>:"controlMove.vi"("Set"=TRUE, "error in"=w475, "control move in"=w471, "axis in"=w474, "connection ID"=w473) -> ("error out"=w472:errorcluster)  [unwired: 3 in, 3 out]
              }
              frame True {
                n229 = call <userlib>:"controlOutput.vi"("error in"=w486, "axis in"=w485, "connection ID"=w484) -> ("error out"=w483:errorcluster, "enable output out"=w482:bool, "axis out"=w479:u8, "connection ID"=w480:refnum<k5>)  [unwired: 5 in]
                n230 = case shown="Faux" w482 {
                  tunnel: w483 -> [w505 w508]
                  tunnel: [w504 w508] -> w481
                  tunnel: w480 -> [w503 w507]
                  tunnel: w479 -> [w502 w506]
                  tunnel: [w501 w507] -> w478
                  tunnel: [w500 w506] -> w477
                  frame False {
                    w499 = TRUE ("Set")
                    n231 = call <userlib>:"controlOutput.vi"("Set"=w499, "error in"=w505, "enable output in"=w499, "axis in"=w502, "connection ID"=w503) -> ("error out"=w504:errorcluster, "axis out"=w500:u8, "connection ID"=w501:refnum<k5>)  [unwired: 3 in, 1 out]
                  }
                  frame True {
                  }
                }
                n232 = call <userlib>:"controlTargetPosition.vi"("error in"=w481, "axis in"=w477, "connection ID"=w478) -> ("error out"=w496:errorcluster, "Target Position out"=w489:dbl, "axis out"=w495:u8, "connection ID"=w494:refnum<k5>)  [unwired: 5 in]
                n233 = call <userlib>:"controlTargetPosition.vi"("Set"=TRUE, "error in"=w496, "Target Position in"=w489, "axis in"=w495, "connection ID"=w494) -> ("error out"=w492:errorcluster, "Target Position out"=w488:dbl, "axis out"=w490:u8, "connection ID"=w491:refnum<k5>)  [unwired: 3 in]
                n234 = local write "Target 2"(w488) -> ()
                n235 = call <userlib>:"controlMove.vi"("Set"=TRUE, "error in"=w492, "control move in"=w497, "axis in"=w490, "connection ID"=w491) -> ("error out"=w487:errorcluster)  [unwired: 3 in, 3 out]
              }
            }
          }
          event "Ctrl 3": Value Change {
            n236 = event-data() -> ("NewVal"=w513:bool)  [unwired: 1 in]
            n237 = local read "ConnID"() -> (w511:refnum<k5>)
            n238 = local read "axis3"() -> (w512:u8)
            n239 = case shown="Vrai" w513 {
              selector: w513 -> [w514 w540]
              tunnel: w511 -> [w516 w527]
              tunnel: w512 -> [w517 w528]
              tunnel: w510 -> [w518 w529]
              tunnel: [w515 w530] -> w509
              frame False {
                n240 = call <userlib>:"controlMove.vi"("Set"=TRUE, "error in"=w518, "control move in"=w514, "axis in"=w517, "connection ID"=w516) -> ("error out"=w515:errorcluster)  [unwired: 3 in, 3 out]
              }
              frame True {
                n241 = call <userlib>:"controlOutput.vi"("error in"=w529, "axis in"=w528, "connection ID"=w527) -> ("error out"=w526:errorcluster, "enable output out"=w525:bool, "axis out"=w522:u8, "connection ID"=w523:refnum<k5>)  [unwired: 5 in]
                n242 = case shown="Faux" w525 {
                  tunnel: w526 -> [w548 w551]
                  tunnel: [w547 w551] -> w524
                  tunnel: w523 -> [w546 w550]
                  tunnel: w522 -> [w545 w549]
                  tunnel: [w544 w550] -> w521
                  tunnel: [w543 w549] -> w520
                  frame False {
                    w542 = TRUE ("Set")
                    n243 = call <userlib>:"controlOutput.vi"("Set"=w542, "error in"=w548, "enable output in"=w542, "axis in"=w545, "connection ID"=w546) -> ("error out"=w547:errorcluster, "axis out"=w543:u8, "connection ID"=w544:refnum<k5>)  [unwired: 3 in, 1 out]
                  }
                  frame True {
                  }
                }
                n244 = call <userlib>:"controlTargetPosition.vi"("error in"=w524, "axis in"=w520, "connection ID"=w521) -> ("error out"=w539:errorcluster, "Target Position out"=w532:dbl, "axis out"=w538:u8, "connection ID"=w537:refnum<k5>)  [unwired: 5 in]
                n245 = call <userlib>:"controlTargetPosition.vi"("Set"=TRUE, "error in"=w539, "Target Position in"=w532, "axis in"=w538, "connection ID"=w537) -> ("error out"=w535:errorcluster, "Target Position out"=w531:dbl, "axis out"=w533:u8, "connection ID"=w534:refnum<k5>)  [unwired: 3 in]
                n246 = local write "Target 3"(w531) -> ()
                n247 = call <userlib>:"controlMove.vi"("Set"=TRUE, "error in"=w535, "control move in"=w540, "axis in"=w533, "connection ID"=w534) -> ("error out"=w530:errorcluster)  [unwired: 3 in, 3 out]
              }
            }
          }
        }
        n248 = Or(x="Quit", y=w9) -> (x .or. y?=w8:bool)
      }
    }
    frame Error {
    }
  }
  "error out" <- w2
